vi "Error_handler.vi"(0 "error constant":errorcluster) -> ()   [LabVIEW 2018]
uses:
  Global/Global Variables/Data_Display_global.vi
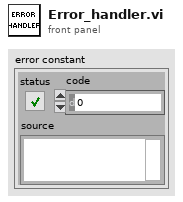
[diagram p1: front panel]
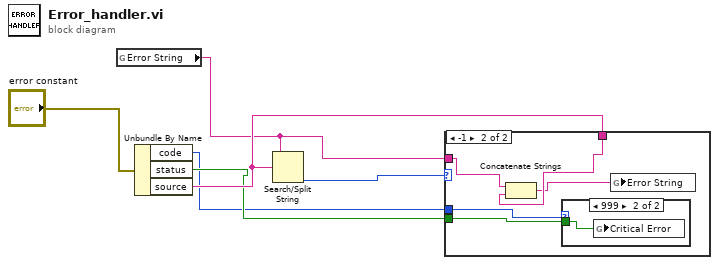
[diagram p0: block diagram]
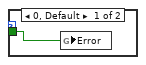
[diagram p3: hidden frame]
diagram:
  n1 = global read "Data_Display_global.vi" "Error String"() -> (w3:string)
  n2 = Unbundle By Name("error constant") -> ("code"=w1:i32, "status"=w2:bool, "source"=w4:string)
  n3 = Search/Split String(string=w3, search string/char (-)=w4) -> (offset of match=w5:i32)  [unwired: 1 in, 2 out]
  n4 = case shown="-1" w5 {
    tunnel: w4 -> [_ w11]
    tunnel: w3 -> [_ w10]
    tunnel: w2 -> [_ w9]
    tunnel: w1 -> [_ w8]
    frame 0, Default {
    }
    frame -1 {
      n5 = Concatenate Strings(w10, w11) -> (w7:string)
      n6 = case shown="999" w8 {
        tunnel: w9 -> [w12 w13]
        frame 0, Default {
          n7 = global write "Data_Display_global.vi" "Error"(w12) -> ()
        }
        frame 999 {
          n8 = global write "Data_Display_global.vi" "Critical Error"(w13) -> ()
        }
      }
      n9 = global write "Data_Display_global.vi" "Error String"(w7) -> ()
    }
  }
